vi "Draw Image to Picture (Greyscale).vi"(7 "Image Draw Offset (Default 0,0)":T1, 8 "error in (no error)":errorcluster, 11 "Greyscale Image Source":T2) -> (0 "error out":errorcluster, 3 "Picture":picture)   [LabVIEW 2020, in "g_ar_toolkit.image.lvlib"]
uses:
  g_ar_toolkit.image.lvlib
  Greyscale Image.ctl
  Image Draw Offset.ctl
  9ae995ca-ccda-485c-89ac-02736fde3e8e.vi
  g_ar_toolkit.common/Module Path.vi
  <vilib>/Utility/error.llb/Error Cluster From Error Code.vi
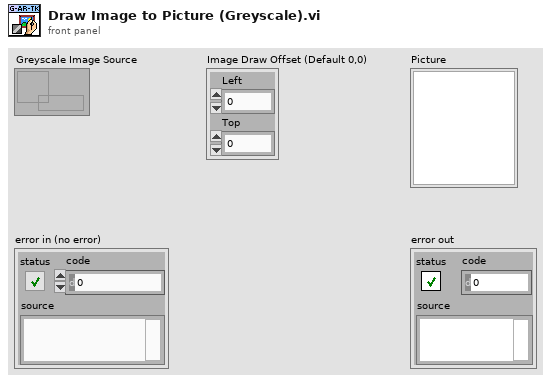
[diagram p1: front panel]
types:
  T1 = typedef "g_ar_toolkit.image.lvlib/Image Draw Offset.ctl" = cluster{"Left":i16, "Top":i16}
  T2 = typedef "g_ar_toolkit.image.lvlib/Greyscale Image.ctl" = refnum<data-value>
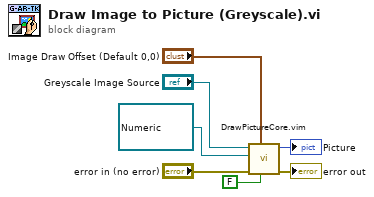
[diagram p0: block diagram]
diagram:
  n1 = call "DrawPictureCore.vim"("HasMask"=FALSE, "Image Draw Offset"="Image Draw Offset (Default 0,0)", "error in (no error)"="error in (no error)", "Image Mask"=refnum<data-value> refnum, "Image Src"="Greyscale Image Source") -> ("error out"=→"error out":errorcluster, "Picture"=→"Picture":picture)  [unwired: 5 in]
